vi "Add Folder Item.vi"(7 "Top-Level? (F)":bool, 8 "error in (no error)":errorcluster, 9 "Order":i32, 11 "Folder":path) -> (0 "error out":errorcluster, 3 "Item":refnum<class "Item.lvclass">)   [LabVIEW 2020, in "VI Properties Editor.lvlib"]
doc: "Initializes class data for <B>Folder</B>."
uses:
  VI Properties Editor.lvlib
  Classes/Item/Item.lvclass
  Classes/Support/Item Type.ctl
  <vilib>/picture/picture.llb/imagedata.ctl
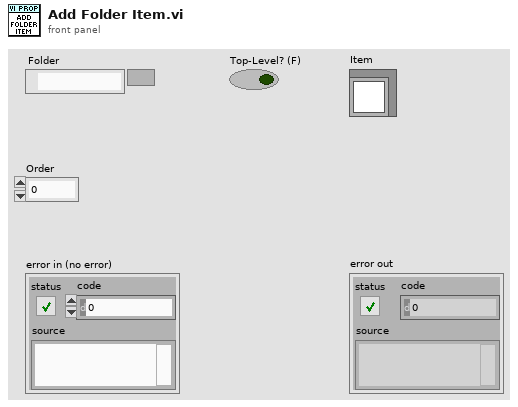
[diagram p1: front panel]
types:
  T1 = typedef "imagedata.ctl" = cluster{"image type":i32, "image depth":i32, "image":u8[], "mask":u8[], "colors":u32[], "Rectangle":cluster{"left":i16, "top":i16, "right":i16, "bottom":i16}}
  T2 = typedef "VI Properties Editor.lvlib/Item Type.ctl" = enum16{"Generic", "VI"}
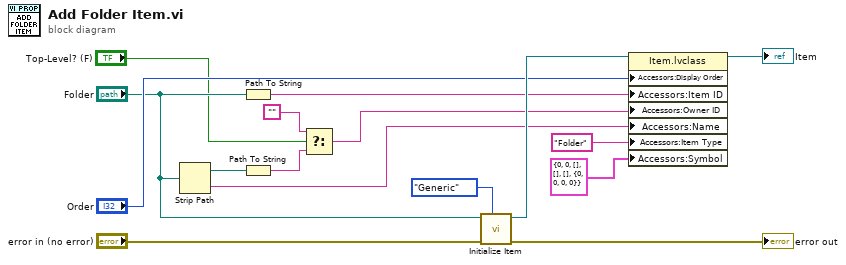
[diagram p0: block diagram]
diagram:
  n1 = Strip Path(path="Folder") -> (stripped path=w5:path, name=w11:string)
  n2 = Path To String(path="Folder") -> (string=w7:string)
  n3 = Path To String(path=w5) -> (string=w4:string)
  n4 = Select(t="", s="Top-Level? (F)", f=w4) -> (s? t:f=w1:string)
  n5 = call "Initialize Item.vi"("Item Type"=Item_Type."Generic", "error in (no error)"="error in (no error)", "Path"="Folder") -> ("error out"=→"error out":errorcluster, "Item"=w15:refnum<class "Item.lvclass">)  [unwired: 7 in]
  n6 = property class="Item.lvclass"(reference=w15, "Accessors:Display Order"="Order", "Accessors:Item ID"=w7, "Accessors:Owner ID"=w1, "Accessors:Name"=w11, "Accessors:Item Type"="Folder" ("Item Type"), "Accessors:Symbol"=T1 {"image type"=0, "image depth"=0, "image"=[], "mask"=[], "colors"=[], "Rectangle"={"left"=0, "top"=0, "right"=0, "bottom"=0}} ("image data")) -> (reference out=→"Item":refnum<class "Item.lvclass">)  [unwired: 1 in, 1 out]
